vi "polar2cartesian.vi"(2 "Range":u16, 3 "Angle":i16) -> (0 "y":i16, 1 "x":i16)   [LabVIEW 2010]
doc: "polar2cartesian.vi converts polar coordinates to cartesian coordinates using a lookup table.\n\n<b>Inputs</b>\nAngle - angle in integer degrees from [-90,90).\nRange - range to point\n\n<b>Outputs</b>\nx - x position of point\ny - y position of point"
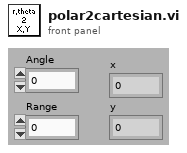
[diagram p1: front panel]
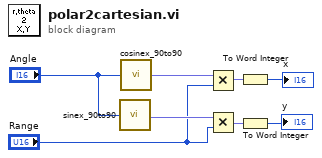
[diagram p0: block diagram]
diagram:
  n1 = call "sinex_90to90.vi"("theta"="Angle") -> ("Numeric"=w7:fxp<+/-,16,1>)
  n2 = call "cosinex_90to90.vi"("theta"="Angle") -> ("Numeric"=w6:fxp<+/-,16,1>)
  n3 = Multiply(x=w6, y="Range") -> (x*y=w4:fxp<+/-,32,17>)
  n4 = Multiply(x=w7, y="Range") -> (x*y=w2:fxp<+/-,32,17>)
  n5 = To Word Integer(number=w4) -> (16bit integer=→"x":i16)
  n6 = To Word Integer(number=w2) -> (16bit integer=→"y":i16)
